vi "test_read-nmea_file.vi"() -> ()   [LabVIEW 2019]
panel:
  out "XY Graph":cluster{"X":dbl, "Y":dbl}[](graph)
  out "array":string[](array[string])
  out "output string":string
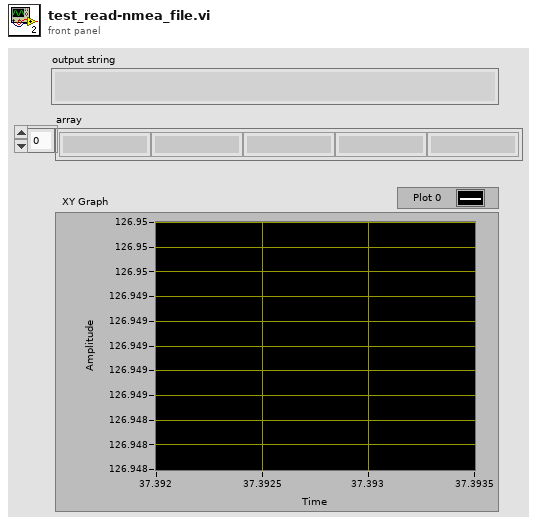
[diagram p1: front panel]
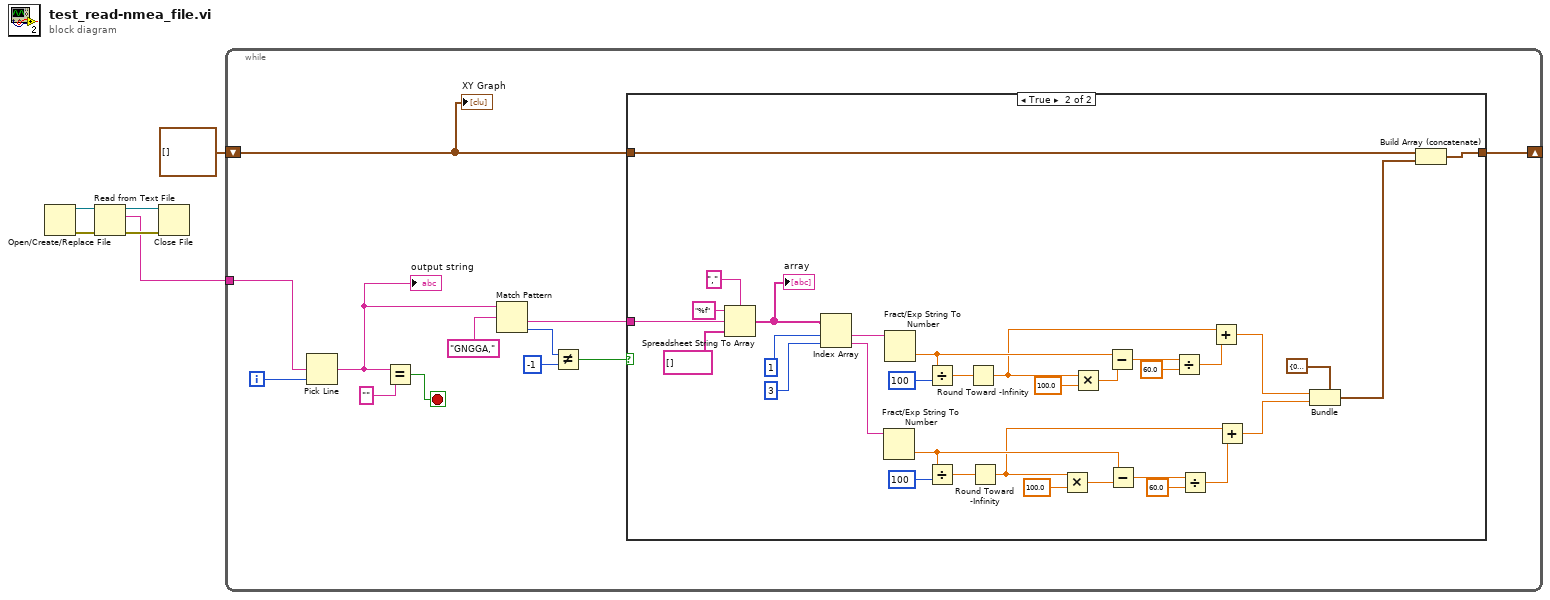
[diagram p0: block diagram]
diagram:
  n1 = Open/Create/Replace File() -> (refnum out=w6:refnum<file>, error out=w4:errorcluster)  [unwired: 6 in, 1 out]
  n2 = Read from Text File(file (use dialog)=w6, error in=w4) -> (refnum out=w5:refnum<file>, text=w2:string, error out=w3:errorcluster)  [unwired: 2 in, 1 out]
  n3 = Close File(refnum=w5, error in=w3) -> ()  [unwired: 2 out]
  n4 = while {
    tunnel: w2 -> [w18]
    shift-right: [w8] -> _
    shift-left: cluster{"lat":dbl, "lon":dbl}[] [] -> [w7]
    i -> [w17]
    stop <- w15 stop-if-true
    n5 = Pick Line(multi-line string=w18, line index=w17) -> (output string=w14:string)  [unwired: 1 in]
    "output string" <- w14
    n6 = Equal?(x=w14, y="") -> (x = y?=w15:bool)
    n7 = Match Pattern(string=w14, regular expression="GNGGA,") -> (after substring=w12:string, offset past match=w11:i32)  [unwired: 1 in, 2 out]
    n8 = Not Equal?(x=w11, y=-1) -> (x != y?=w9:bool)
    n9 = case shown="True" w9 {
      tunnel: w12 -> [_ w50]
      tunnel: w7 -> [w19 w21]
      tunnel: [w19 w20] -> w8
      frame False {
      }
      frame True {
        n10 = Spreadsheet String To Array(delimiter (Tab)=",", format string="%f", spreadsheet string=w50, array type (2D Dbl)=string[] []) -> (array=w25:string[])
        "array" <- w25
        n11 = Index Array(array=w25, index #1=1 ("index"), index #2=3 ("index")) -> (element #1=w38:string, element #2=w37:string)
        n12 = Fract/Exp String To Number(string=w37) -> (number=w39:dbl)  [unwired: 3 in, 1 out]
        n13 = Fract/Exp String To Number(string=w38) -> (number=w40:dbl)  [unwired: 3 in, 1 out]
        n14 = Divide(x=w40, y=100) -> (x/y=w44:dbl)
        n15 = Divide(x=w39, y=100) -> (x/y=w41:dbl)
        n16 = Round Toward -Infinity(1:w44) -> (0:w31:dbl)
        n17 = Round Toward -Infinity(1:w41) -> (0:w29:dbl)
        n18 = Multiply(x=w29, y=100.0) -> (x*y=w42:dbl)
        n19 = Multiply(x=w31, y=100.0) -> (x*y=w43:dbl)
        n20 = Subtract(x=w40, y=w43) -> (x-y=w36:dbl)
        n21 = Subtract(x=w39, y=w42) -> (x-y=w33:dbl)
        n22 = Divide(x=w36, y=60.0) -> (x/y=w32:dbl)
        n23 = Divide(x=w33, y=60.0) -> (x/y=w30:dbl)
        n24 = Add(x=w31, y=w32) -> (x+y=w28:dbl)
        n25 = Add(x=w29, y=w30) -> (x+y=w27:dbl)
        n26 = Bundle(cluster=cluster{"lat":dbl, "lon":dbl} {"lat"=0.0, "lon"=0.0} ("클러스터"), "lat"=w28, "lon"=w27) -> (w22:cluster{"lat":dbl, "lon":dbl})
        n27 = Build Array (concatenate)(w21, w22) -> (w20:cluster{"lat":dbl, "lon":dbl}[])
      }
    }
    "XY Graph" <- w7
  }
